vi "fileRead.vi"() -> ()   [LabVIEW 2014]
panel:
  out "XY Graph":cluster{i32, dbl}[](graph)
  out "Header Line":string
  out "File I/O Error":errorcluster
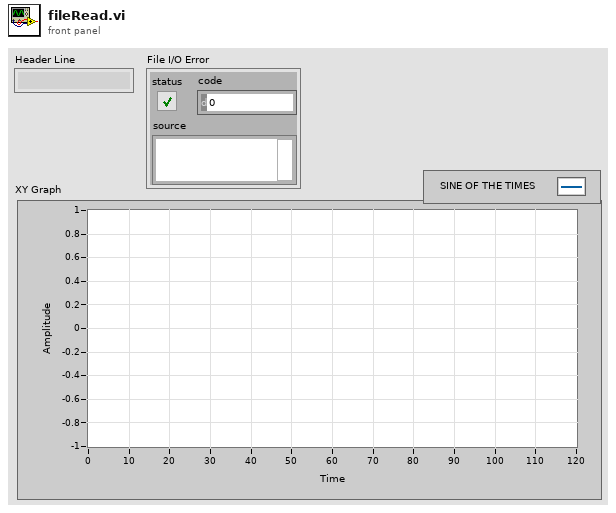
[diagram p1: front panel]
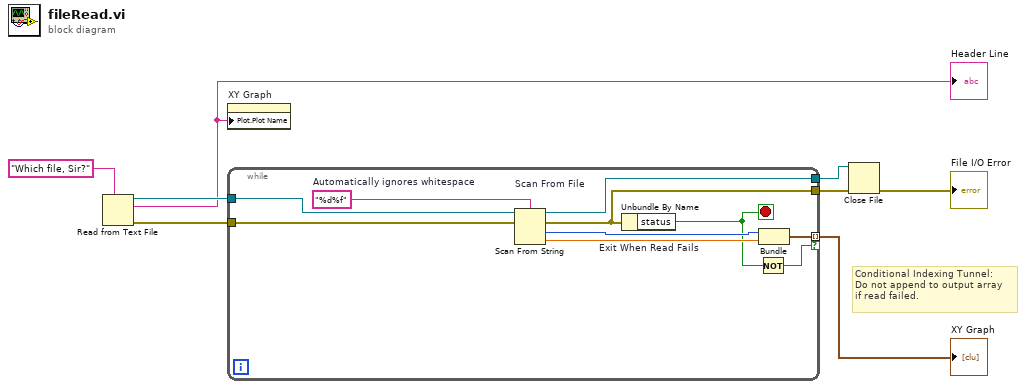
[diagram p0: block diagram]
diagram:
  # "Conditional Indexing Tunnel:\nDo not append to output array\nif read failed."
  n1 = Read from Text File(prompt (Open existing file)="Which file, Sir?") -> (refnum out=w5:refnum<file>, text=w2:string, error out=w4:errorcluster)  [unwired: 3 in, 1 out]
  "Header Line" <- w2
  n2 = property on="XY Graph" class="XYGraph (strict)"("Plot.Plot Name"=w2) -> ()  [unwired: 2 in, 2 out]
  n3 = while {
    tunnel: w4 -> [w18]
    tunnel: [w11] -> w8
    tunnel: w5 -> [w17]
    tunnel: [w16] -> w7
    tunnel: [w12] -> w3 mode=indexing if=w9
    stop <- w10 stop-if-true
    w15 = "%d%f"  # Automatically ignores whitespace
    n4 = Scan From String "Scan From File"(w15, w17, w18) -> (w16:refnum<file>, w11:errorcluster, output 1=w14:i32, output 2=w13:dbl)  [unwired: 2 in]
    n5 = Unbundle By Name "Exit When Read Fails"(w11) -> ("status"=w10:bool)
    n6 = Not(x=w10) -> (.not. x?=w9:bool)
    n7 = Bundle(w14, w13) -> (w12:cluster{i32, dbl})  [unwired: 1 in]
  }
  "XY Graph" <- w3
  n8 = Close File(refnum=w7, error in=w8) -> (error out=→"File I/O Error":errorcluster)  [unwired: 1 out]
